vi "Untitled 1.vi"() -> ()   [LabVIEW 2020]
panel:
  in  "stop":bool
  in  "Slide":dbl(slide) min=0.0 max=10000.0 scale=0.0..10000.0
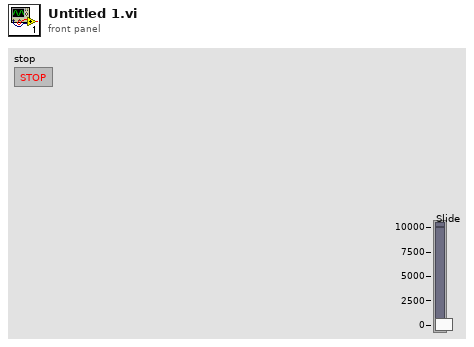
[diagram p1: front panel]
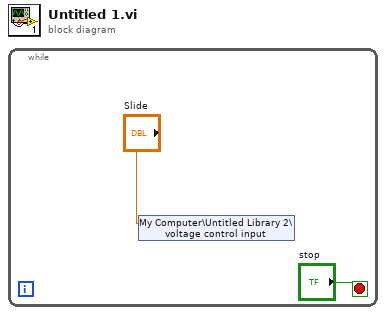
[diagram p0: block diagram]
diagram:
  n1 = while {
    stop <- "stop" stop-if-true
    n2 = shared-variable "My Computer\\Untitled Library 2\\voltage control input"("Slide") -> ()  [unwired: 1 in, 1 out]
  }
